vi "CRYPlot XY Graph.vi"(6 "sOption":string, 7 "pGraph VI In":refnum<vi>, 8 "sType":string, 9 "Flattened Property":string, 10 "Flattened Scale Property":string, 11 "Selected Rows In":i32[](array[numeric])) -> (0 "Color Info":u32[](array[numeric]), 1 "Curve Name":string[](array[string]), 2 "All Rows Out":i32[](array[numeric]), 3 "ItemSyms":i32[](array[numeric]))   [LabVIEW 2013]
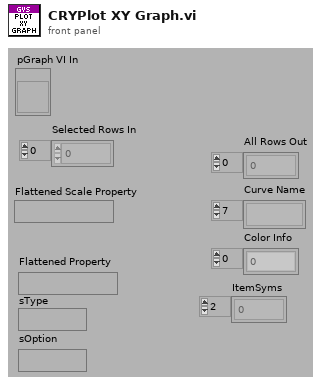
[diagram p1: front panel]
types:
  T1 = cluster{"Color":u32, "Interpolation":u8, "Point Style":u8, "Line Style":u8, "Point Color":u32, "Line Width":u8, "Bar Plot Style":u8, "Fill To":i16}[]
  T2 = typedef "CRYData Cluster.ctl" = cluster{"Name":string, "Curve":cluster{"x":dbl, "y":dbl, "z":dbl}[], "X data":u16, "Y data":u16, "Z data":u16, "X axis":u16, "Y axis":u16, "Z axis":u16, "X unit":string, "Y unit":string, "Z unit":string, "X dB ref":dbl, "Y dB ref":dbl, "Z dB ref":dbl, "single val":bool, "protected":bool, "display X":bool, "display Y":bool, "display Z":bool, "Test Info":string, "Step No.":i32, "Plot Settings":cluster{"Color":u32, "Interpolation":u8, "Point Style":u8, "Line Style":u8, "Point Color":u32, "Line Width":u8, "Bar Plot Style":u8, "Fill To":i16}, "AutoProtect":bool}
  T3 = cluster{"Color":u32, "Interpolation":u8, "Point Style":u8, "Line Style":u8, "Point Color":u32, "Line Width":u8, "Bar Plot Style":u8, "Fill To":i16}
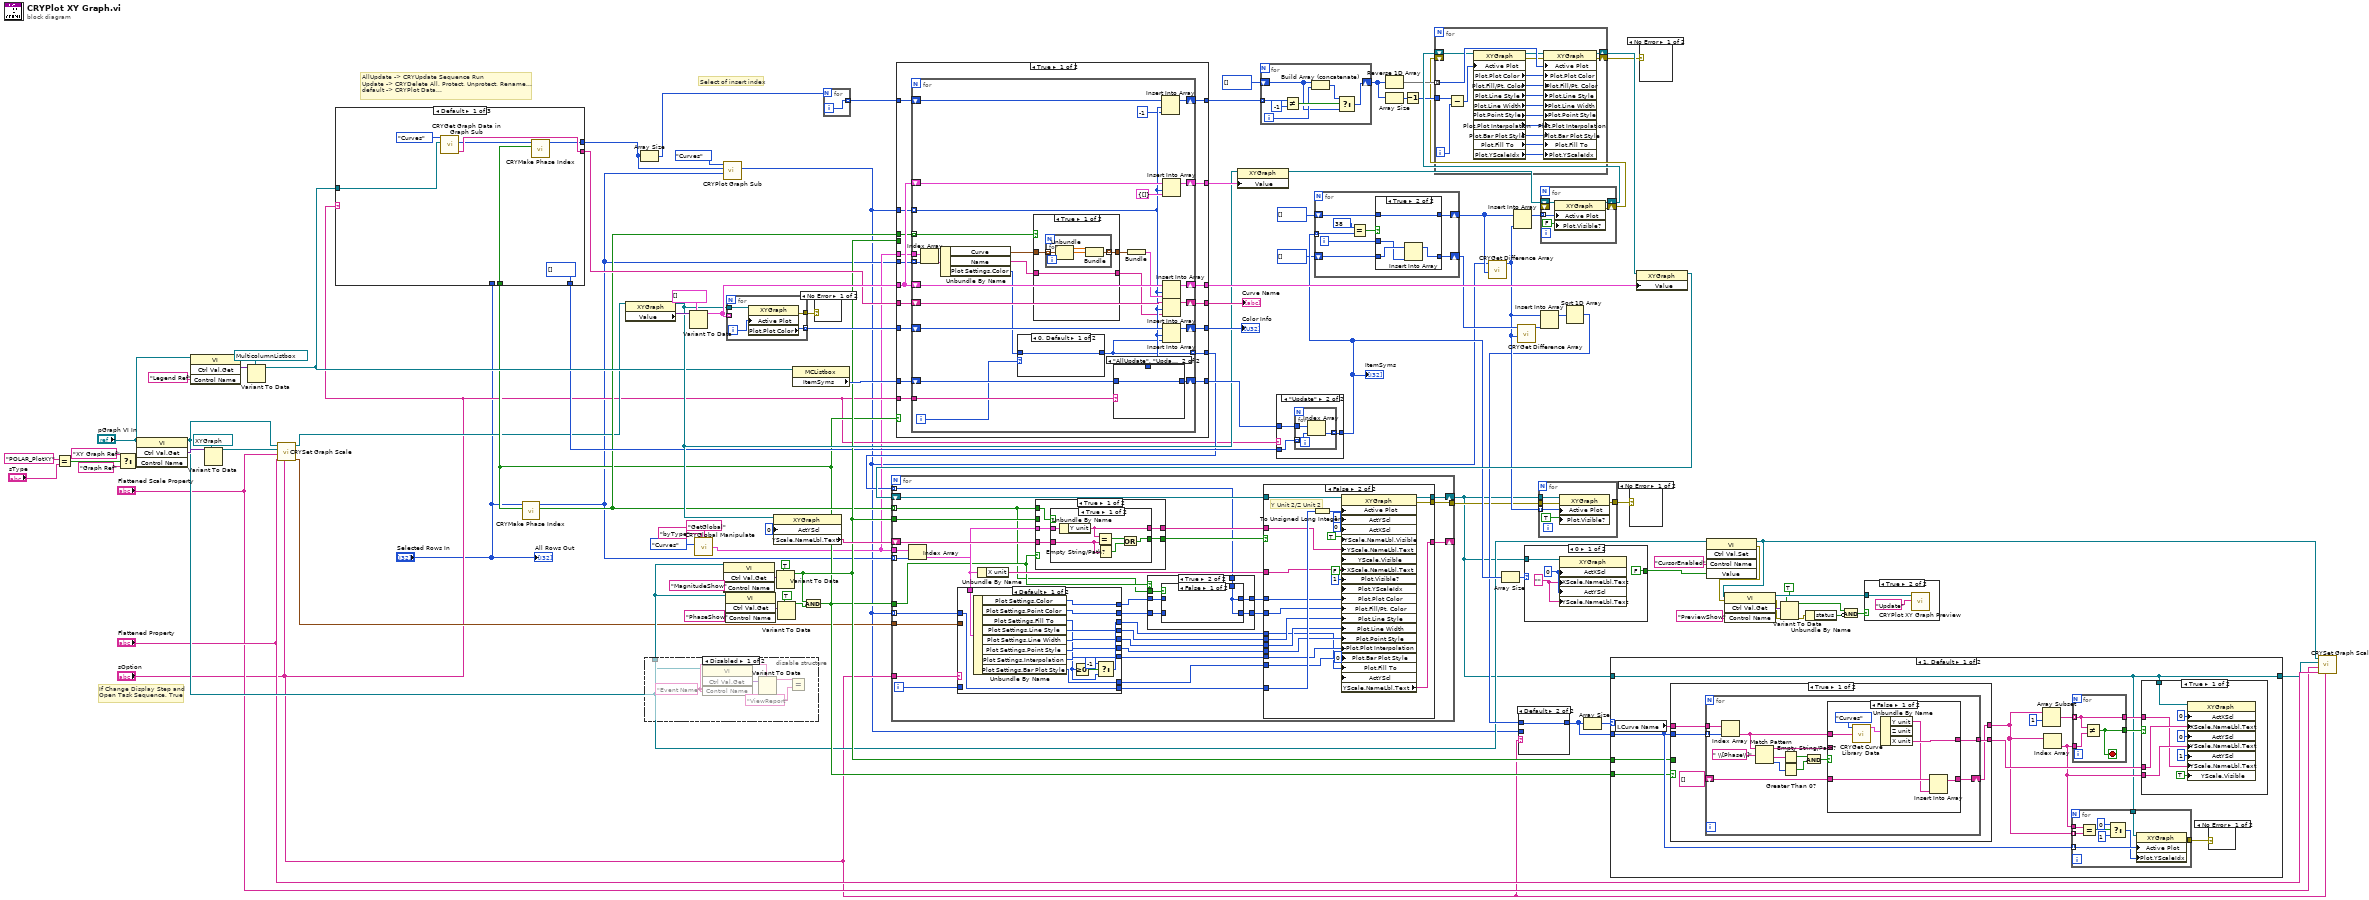
[diagram p0: block diagram]
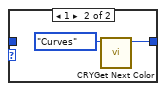
[diagram p5: hidden frame]
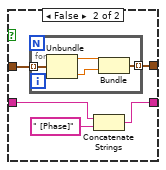
[diagram p6: hidden frame]
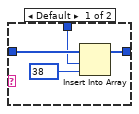
[diagram p7: hidden frame]
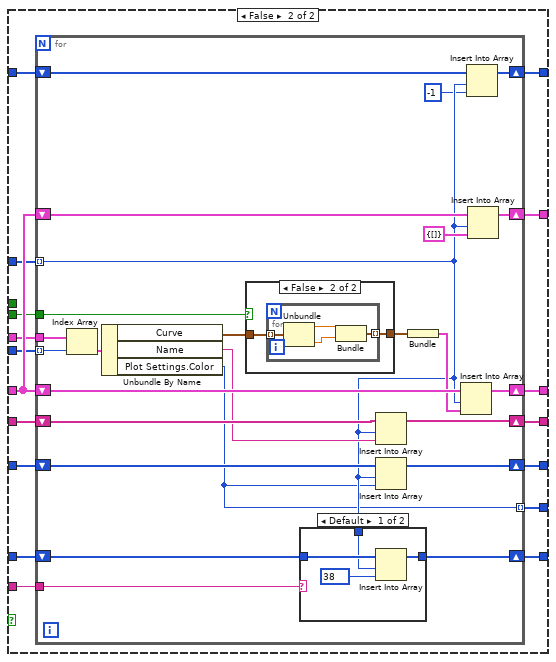
[diagram p8: hidden frame]
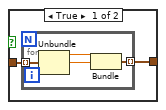
[diagram p9: hidden frame]
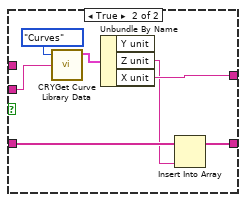
[diagram p14: hidden frame]
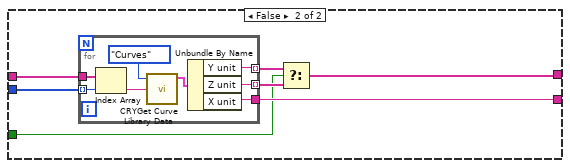
[diagram p15: hidden frame]
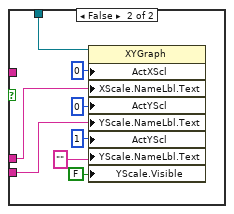
[diagram p16: hidden frame]
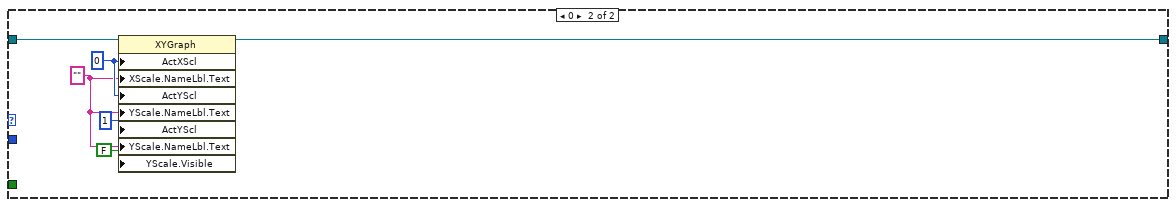
[diagram p17: hidden frame]
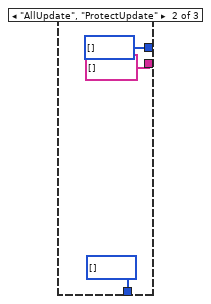
[diagram p19: hidden frame]
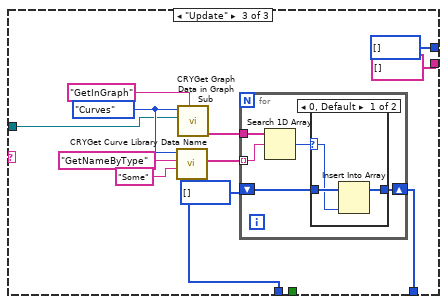
[diagram p20: hidden frame]
diagram:
  # "AllUpdate -> CRYUpdate Sequence Run\nUpdate -> CRYDelete All, Protect, Unprotect, Rename...\ndefault -> CRYPlot Data..."
  # "Select of insert index"
  # "If Change Display Step and \nOpen Task Sequence, True"
  n1 = Equal?(x="POLAR_PlotXY" ("Control Name"), y="sType") -> (x = y?=w33:bool)
  n2 = Select(t="XY Graph Ref", s=w33, f="Graph Ref" ("Control Name")) -> (s? t:f=w30:string)
  n3 = invoke class="VI" method="Ctrl Val.Get"(reference="pGraph VI In", "Control Name"=w30) -> (reference out=w19:refnum<vi>, "Get Control Value Variant"=w40:variant)  [unwired: 2 in, 2 out]
  n4 = invoke class="VI" method="Ctrl Val.Get"(reference="pGraph VI In", "Control Name"="Legend Ref") -> ("Get Control Value Variant"=w38:variant)  [unwired: 2 in, 3 out]
  n5 = Variant To Data(type=refnum<vi> refnum ("XY Graph"), Variant=w40) -> (data=w18:refnum<vi>)  [unwired: 1 in, 1 out]
  n6 = Variant To Data(type=refnum<vi> refnum ("GMListbox"), Variant=w38) -> (data=w35:refnum<vi>)  [unwired: 1 in, 1 out]
  n7 = call "CRYSet Graph Scale.vi"("sOption"="sOption", "Flattened Property"="Flattened Property", "Flattened Scale Property"="Flattened Scale Property", "pGraph In"=w18, "pGraph VI In"=w19) -> ("Plot Settings"=w16:T1, "pGraph Out"=w17:refnum<vi>)  [unwired: 5 in]
  n8 = property class="XYGraph"(reference=w17) -> (reference out=w59:refnum<vi>, "Value"=w97:variant)  [unwired: 1 in, 1 out]
  n9 = disable-structure shown="Disabled" {
    disable-tunnel: w19 -> [w101 _]
    frame Disabled {
      w102 = "Event Name" ("Control Name")
      n10 = invoke class="VI" method="Ctrl Val.Get"(reference=w101, "Control Name"=w102) -> ("Get Control Value Variant"=w105:variant)  [unwired: 2 in, 3 out]
      n11 = Variant To Data(type=w102, Variant=w105) -> (data=w104:string)  [unwired: 1 in, 1 out]
      n12 = Equal?(x=w104, y="ViewReport" ("regular expression")) -> ()  [unwired: 1 out]
    }
    frame Enabled {
    }
  }
  n13 = Variant To Data(type=cluster{cluster{"x":dbl, "z":dbl}[]}[] [], Variant=w97) -> (data=w96:cluster{cluster{"x":dbl, "z":dbl}[]}[])  [unwired: 1 in, 1 out]
  n14 = call "CRYGlobal Manipulate.vi"("Type"=enum16{"Curves", "Values", "Results", "WFM"}."Curves", "sOption"="byType", "sAction"="GetGlobal") -> ("Curves Out"=w6:T2[])  [unwired: 6 in, 6 out]
  n15 = invoke class="VI" method="Ctrl Val.Get"(reference=w19, "Control Name"="MagnitudeShow") -> ("Get Control Value Variant"=w69:variant)  [unwired: 2 in, 3 out]
  n16 = invoke class="VI" method="Ctrl Val.Get"(reference=w19, "Control Name"="PhaseShow") -> ("Get Control Value Variant"=w27:variant)  [unwired: 2 in, 3 out]
  n17 = for {
    tunnel: w96 -> [_] mode=indexing
    tunnel: w59 -> [w109]
    tunnel: [w108] -> w95 mode=indexing
    tunnel: [w106] -> w42
    i -> [w107]
    n18 = property class="XYGraph"(reference=w109, "Active Plot"=w107) -> (error out=w106:errorcluster, "Plot.Plot Color"=w108:u32)  [unwired: 1 in, 1 out]
  }
  n19 = property class="XYGraph"(reference=w59, "ActYScl"=0 ("Active Y Scale")) -> ("YScale.NameLbl.Text"=w58:string)  [unwired: 1 in, 2 out]
  n20 = Variant To Data(type=TRUE, Variant=w69) -> (data=w25:bool)  [unwired: 1 in, 1 out]
  n21 = Variant To Data(type=TRUE, Variant=w27) -> (data=w24:bool)  [unwired: 1 in, 1 out]
  n22 = property class="MCListbox"(reference=w35) -> ("ItemSyms"=w87:i32[])  [unwired: 1 in, 2 out]
  n23 = And(x=w25, y=w24) -> (x .and. y?=w20:bool)
  n24 = case shown="Default" "sOption" {
    tunnel: [w116 string[] [] ("Names Out") string[] [] ("Names Out")] -> w92
    tunnel: [w112 i32[] [] ("Rows") i32[] [] ("Rows")] -> w3
    tunnel: "Selected Rows In" -> [_ _ w125]
    tunnel: [i32[] [] i32[] [] w121] -> w23
    tunnel: w35 -> [w113 _ w120]
    tunnel: w20 -> [w111 _ _]
    frame Default {
      n25 = call "CRYGet Graph Data in Graph Sub.vi"("Legend Refnum"=w113, "Type In"=enum16{"Curves", "Values", "Results", "WFM"}."Curves" ("Type")) -> ("Names Out"=w116:string[], "Rows"=w110:i32[])  [unwired: 5 in, 3 out]
      n26 = call "CRYMake Phase Index.vi"("Mag_Phase Flag"=w111, "Selected Rows In"=w110) -> ("Selected Rows Out"=w112:i32[])  [unwired: 8 in, 1 out]
    }
    frame "AllUpdate", "ProtectUpdate" {
    }
    frame "Update" {
      w128 = enum16{"Curves", "Values", "Results", "WFM"}."Curves" ("Type")
      n27 = call "CRYGet Curve Library Data Name.vi"("nData"=w125, "sOption"="Some", "sAction"="GetNameByType", "Type"=w128) -> ("sNames"=w123:string[])  [unwired: 4 in, 3 out]
      n28 = call "CRYGet Graph Data in Graph Sub.vi"("sOption"="GetInGraph", "Legend Refnum"=w120, "Type In"=w128) -> ("Names Out"=w124:string[])  [unwired: 4 in, 4 out]
      n29 = for {
        tunnel: w124 -> [w133]
        tunnel: w123 -> [w132] mode=indexing
        shift-right: [w134] -> w121
        shift-left: i32[] [] -> [w135]
        n30 = Search 1D Array(1D array=w133, element=w132) -> (index of element=w136:i32)  [unwired: 1 in]
        n31 = case shown="0, Default" w136 {
          selector: w136 -> [w137 _]
          tunnel: w135 -> [w139 w140]
          tunnel: [w138 w140] -> w134
          frame 0, Default {
            n32 = Insert Into Array(array=w139, new element=w137) -> (w138:i32[])  [unwired: 1 in]
          }
          frame -1 {
          }
        }
      }
    }
  }
  n33 = call "CRYMake Phase Index.vi"("Mag_Phase Flag"=w20, "Selected Rows In"="Selected Rows In") -> ("Mag_Phase"=w22:bool[], "Selected Rows Out"=w2:i32[])  [unwired: 8 in]
  n34 = Array Size(array=w3) -> (size(s)=w65:i32)
  n35 = call "CRYPlot Graph Sub.vi"("nData2 In"=w2, "nData1 In"=w3, "Type"=enum16{"Curves", "Values", "Results", "WFM"}."Curves") -> ("nData Out"=w1:i32[])  [unwired: 8 in]
  n36 = case shown="No Error" w42 {
    frame No Error {
    }
    frame Error {
    }
  }
  n37 = for {
    N: w65 -> [_]
    tunnel: [w141] -> w85 mode=indexing
    i -> [w141]
  }
  n38 = case shown="True" w20 {
    tunnel: w96 -> [w158 w227]
    tunnel: w95 -> [w157 w226]
    tunnel: [w156 w225] -> w94
    tunnel: w92 -> [w155 w224]
    tunnel: [w154 w223] -> w89
    tunnel: [w153 w222] -> w88
    tunnel: w87 -> [w152 w221]
    tunnel: w85 -> [w151 w220]
    tunnel: [w150 w219] -> w84
    tunnel: [w149 w218] -> w75
    tunnel: [w148 w217] -> w62
    tunnel: w6 -> [w147 w216]
    tunnel: w2 -> [w146 w215]
    tunnel: w1 -> [w145 w214]
    tunnel: "sOption" -> [w144 w213]
    tunnel: w25 -> [_ w212]
    tunnel: w22 -> [w143 _]
    tunnel: [w142 w211] -> w21
    frame True {
      n39 = for {
        tunnel: w147 -> [w186]
        tunnel: w146 -> [w183] mode=indexing
        shift-right: [w184] -> w154
        shift-left: w158 -> [w185]
        tunnel: w145 -> [w167] mode=indexing
        shift-right: [w175] -> w156
        shift-left: w155 -> [w178]
        shift-right: [w176] -> w149
        shift-left: w157 -> [w177]
        shift-right: [w173] -> w153
        shift-left: w158 -> [w172]
        shift-right: [w170] -> w148
        shift-left: w152 -> [w171]
        shift-right: [w168] -> w150
        shift-left: w151 -> [w169]
        tunnel: w144 -> [w165]
        tunnel: w143 -> [w164] mode=indexing
        tunnel: [w159] -> w142 mode=indexing
        i -> [w161]
        n40 = Index Array(array=w186, index=w183) -> (element=w180:T2)
        n41 = Unbundle By Name(w180) -> ("Curve"=w181:cluster{"x":dbl, "y":dbl, "z":dbl}[], "Name"=w163:string, "Plot Settings.Color"=w160:u32)
        n42 = case shown="0, Default" w161 {
          tunnel: w160 -> [w187 _]
          tunnel: [w187 w188] -> w159
          frame 0, Default {
          }
          frame 1 {
            n43 = call "CRYGet Next Color.vi"("Type"=enum16{"Curves", "Values", "Results", "WFM"}."Curves") -> ("Color"=w188:u32)  [unwired: 10 out]
          }
        }
        n44 = case shown="True" w164 {
          tunnel: [w192 w201] -> w182
          tunnel: w181 -> [w191 w200]
          tunnel: w163 -> [w190 w199]
          tunnel: [w190 w197] -> w162
          frame True {
            n45 = for {
              tunnel: w191 -> [w196] mode=indexing
              tunnel: [w195] -> w192 mode=indexing
              n46 = Unbundle(w196) -> ("x"=w194:dbl, "y"=w193:dbl)  [unwired: 1 out]
              n47 = Bundle("x"=w194, "y"=w193) -> (w195:cluster{"x":dbl, "y":dbl})  [unwired: 1 out]
            }
          }
          frame False {
            n48 = for {
              tunnel: w200 -> [w205] mode=indexing
              tunnel: [w204] -> w201 mode=indexing
              n49 = Unbundle(w205) -> ("x"=w203:dbl, "z"=w202:dbl)  [unwired: 1 out]
              n50 = Bundle("x"=w203, "z"=w202) -> (w204:cluster{"x":dbl, "z":dbl})  [unwired: 1 out]
            }
            n51 = Concatenate Strings(w199, " [Phase]" ("regular expression")) -> (w197:string)
          }
        }
        n52 = case shown="\"AllUpdate\", \"Update\"" w165 {
          tunnel: w171 -> [w209 w210]
          tunnel: [w208 w210] -> w170
          tunnel: w167 -> [w206 _]
          frame Default {
            n53 = Insert Into Array(array=w209, index=w206, new element=38) -> (w208:i32[])
          }
          frame "AllUpdate", "Update" {
          }
        }
        n54 = Bundle(w182) -> (w179:cluster{cluster{"x":dbl, "z":dbl}[]})  [unwired: 1 in]
        n55 = Insert Into Array(array=w169, index=w167, new element=-1 ("new element/subarray")) -> (w168:i32[])
        n56 = Insert Into Array(array=w172, index=w167, new element=cluster{cluster{"x":dbl, "y":dbl}[]} {[]} ("output cluster")) -> (w173:cluster{cluster{"x":dbl, "z":dbl}[]}[])
        n57 = Insert Into Array(array=w185, index=w167, new element=w179) -> (w184:cluster{cluster{"x":dbl, "z":dbl}[]}[])
        n58 = Insert Into Array(array=w178, index=w167, new element=w162) -> (w175:string[])
        n59 = Insert Into Array(array=w177, index=w167, new element=w159) -> (w176:u32[])
      }
    }
    frame False {
      n60 = for {
        tunnel: w216 -> [w252]
        tunnel: w215 -> [w249] mode=indexing
        shift-right: [w250] -> w223
        shift-left: w227 -> [w251]
        tunnel: w214 -> [w232] mode=indexing
        shift-right: [w240] -> w225
        shift-left: w224 -> [w244]
        shift-right: [w241] -> w218
        shift-left: w226 -> [w242]
        shift-right: [w238] -> w222
        shift-left: w227 -> [w237]
        shift-right: [w235] -> w217
        shift-left: w221 -> [w236]
        shift-right: [w233] -> w219
        shift-left: w220 -> [w234]
        tunnel: w213 -> [w230]
        tunnel: w212 -> [w229]
        tunnel: [w228] -> w211 mode=indexing
        n61 = Index Array(array=w252, index=w249) -> (element=w246:T2)
        n62 = Unbundle By Name(w246) -> ("Curve"=w247:cluster{"x":dbl, "y":dbl, "z":dbl}[], "Name"=w243:string, "Plot Settings.Color"=w228:u32)
        n63 = case shown="False" w229 {
          tunnel: [w254 w260] -> w248
          tunnel: w247 -> [w253 w259]
          frame True {
            n64 = for {
              tunnel: w253 -> [w258] mode=indexing
              tunnel: [w257] -> w254 mode=indexing
              n65 = Unbundle(w258) -> ("x"=w256:dbl, "y"=w255:dbl)  [unwired: 1 out]
              n66 = Bundle("x"=w256, "y"=w255) -> (w257:cluster{"x":dbl, "y":dbl})  [unwired: 1 out]
            }
          }
          frame False {
            n67 = for {
              tunnel: w259 -> [w264] mode=indexing
              tunnel: [w263] -> w260 mode=indexing
              n68 = Unbundle(w264) -> ("x"=w262:dbl, "z"=w261:dbl)  [unwired: 1 out]
              n69 = Bundle("x"=w262, "z"=w261) -> (w263:cluster{"x":dbl, "z":dbl})  [unwired: 1 out]
            }
          }
        }
        n70 = case shown="Default" w230 {
          tunnel: w236 -> [w268 w269]
          tunnel: [w267 w269] -> w235
          tunnel: w232 -> [w265 _]
          frame Default {
            n71 = Insert Into Array(array=w268, index=w265, new element=38) -> (w267:i32[])
          }
          frame "AllUpdate", "Update" {
          }
        }
        n72 = Insert Into Array(array=w244, index=w232, new element=w243) -> (w240:string[])
        n73 = Insert Into Array(array=w242, index=w232, new element=w228) -> (w241:u32[])
        n74 = Bundle(w248) -> (w245:cluster{cluster{"x":dbl, "z":dbl}[]})  [unwired: 1 in]
        n75 = Insert Into Array(array=w251, index=w232, new element=w245) -> (w250:cluster{cluster{"x":dbl, "z":dbl}[]}[])
        n76 = Insert Into Array(array=w234, index=w232, new element=-1 ("new element/subarray")) -> (w233:i32[])
        n77 = Insert Into Array(array=w237, index=w232, new element=cluster{cluster{"x":dbl, "y":dbl}[]} {[]} ("output cluster")) -> (w238:cluster{cluster{"x":dbl, "z":dbl}[]}[])
      }
    }
  }
  "Curve Name" <- w94
  "Color Info" <- w75
  n78 = property class="XYGraph"(reference=w59, "Value"=w88) -> (reference out=w90:refnum<vi>)  [unwired: 1 in, 1 out]
  n79 = for {
    tunnel: w84 -> [w276] mode=indexing
    shift-right: [w272] -> w79
    shift-left: i32[] [] ("Selected Rows In") -> [w270]
    i -> [w271]
    n80 = Not Equal?(x=w276, y=-1) -> (x != y?=w274:bool)
    n81 = Build Array (concatenate)(w270, w271) -> (w273:i32[])
    n82 = Select(t=w273, s=w274, f=w270) -> (s? t:f=w272:i32[])
  }
  n83 = case shown="\"Update\"" "sOption" {
    tunnel: w23 -> [_ w279]
    tunnel: w62 -> [w277 w280]
    tunnel: [w277 w278] -> w61
    frame Default {
    }
    frame "Update" {
      n84 = for {
        tunnel: w280 -> [w283]
        tunnel: w279 -> [w282] mode=indexing
        tunnel: [w281] -> w278 mode=indexing
        n85 = Index Array(array=w283, index=w282) -> (element=w281:i32)
      }
    }
  }
  "ItemSyms" <- w61
  n86 = for {
    tunnel: w61 -> [w290] mode=indexing
    shift-right: [w289] -> w63
    shift-left: i32[] [] ("Selected Rows In") -> [w288]
    shift-right: [w284] -> w55
    shift-left: i32[] [] ("Selected Rows In") -> [w285]
    i -> [w287]
    n87 = Equal?(x=38, y=w290) -> (x = y?=w286:bool)
    n88 = case shown="True" w286 {
      tunnel: [w293 w299] -> w289
      tunnel: w288 -> [w294 w299]
      tunnel: w287 -> [w295 w297]
      tunnel: w285 -> [w292 w298]
      tunnel: [w292 w296] -> w284
      frame False {
        n89 = Insert Into Array(array=w294, new element=w295) -> (w293:i32[])  [unwired: 1 in]
      }
      frame True {
        n90 = Insert Into Array(array=w298, new element=w297) -> (w296:i32[])  [unwired: 1 in]
      }
    }
  }
  n91 = Reverse 1D Array(array=w79) -> (reversed array=w80:i32[])
  n92 = Array Size(array=w79) -> (size(s)=w78:i32)
  n93 = Decrement(x=w78) -> (x-1=w77:i32)
  n94 = call "CRYGet Difference Array.vi"("Array 2"=w63, "Array 1"=w1) -> ("Diff Out"=w54:i32[])  [unwired: 8 in, 1 out]
  n95 = Array Size(array=w61) -> (size(s)=w100:i32)
  n96 = Insert Into Array(array=w63, new element=w54) -> (w64:i32[])  [unwired: 1 in]
  n97 = call "CRYGet Difference Array.vi"("Array 2"=w54, "Array 1"=w55) -> ("Diff Out"=w53:i32[])  [unwired: 8 in, 1 out]
  n98 = for {
    shift-right: [w302] -> w82
    shift-left: w90 -> [w304]
    tunnel: w64 -> [w301] mode=indexing
    shift-right: [w300] -> w66
    shift-left: _ -> [_]
    n99 = property class="XYGraph"(reference=w304, "Active Plot"=w301, "Plot.Visible?"=FALSE ("Plot.Visible")) -> (reference out=w302:refnum<vi>, error out=w300:errorcluster)  [unwired: 1 in]
  }
  n100 = for {
    tunnel: w80 -> [w317] mode=indexing
    shift-right: [w315] -> w81
    shift-left: w82 -> [w316]
    tunnel: w77 -> [w312]
    shift-right: [w308] -> w76
    shift-left: w66 -> [_]
    i -> [w311]
    n101 = Subtract(x=w312, y=w311) -> (x-y=w310:i32)
    n102 = property class="XYGraph"(reference=w316, "Active Plot"=w310) -> (reference out=w314:refnum<vi>, error out=w309:errorcluster, "Plot.Plot Color"=w322:u32, "Plot.Fill/Pt. Color"=w321:u32, "Plot.Line Style"=w320:u8, "Plot.Line Width"=w319:u8, "Plot.Point Style"=w318:u8, "Plot.Plot Interpolation"=w313:u8, "Plot.Bar Plot Style"=w307:u8, "Plot.Fill To"=w306:i16, "Plot.YScaleIdx"=w305:u32)  [unwired: 1 in]
    n103 = property class="XYGraph"(reference=w314, error in=w309, "Active Plot"=w317, "Plot.Plot Color"=w322, "Plot.Fill/Pt. Color"=w321, "Plot.Line Style"=w320, "Plot.Line Width"=w319, "Plot.Point Style"=w318, "Plot.Plot Interpolation"=w313, "Plot.Bar Plot Style"=w307, "Plot.Fill To"=w306, "Plot.YScaleIdx"=w305) -> (reference out=w315:refnum<vi>, error out=w308:errorcluster)
  }
  n104 = Insert Into Array(array=w54, new element=w53) -> (w52:i32[])  [unwired: 1 in]
  n105 = Sort 1D Array(array=w52) -> (sorted array=w51:i32[])
  n106 = case shown="Default" "sOption" {
    tunnel: w51 -> [_ w324]
    tunnel: [w323 w324] -> w50
    tunnel: w1 -> [w323 _]
    frame "AllUpdate", "ProtectUpdate", "SepuenceOpen" {
    }
    frame Default {
    }
  }
  n107 = Array Size(array=w50) -> (size(s)=w57:i32)
  n108 = property class="XYGraph"(reference=w81, "Value"=w89) -> (reference out=w93:refnum<vi>)  [unwired: 1 in, 1 out]
  n109 = for {
    tunnel: w2 -> [w354] mode=indexing
    tunnel: w6 -> [w353]
    tunnel: w16 -> [w348]
    tunnel: "sOption" -> [w349]
    tunnel: w25 -> [w338]
    shift-right: [w350] -> w10
    shift-left: w93 -> [w337]
    tunnel: w1 -> [w336] mode=indexing
    shift-right: [w334] -> _
    shift-left: w58 -> [w341]
    tunnel: [w332] -> w43
    tunnel: w22 -> [w326] mode=indexing
    tunnel: w20 -> [w331]
    tunnel: w21 -> [w325] mode=indexing
    i -> [w342]
    n110 = Index Array(array=w353, index=w354) -> (element=w340:T2)
    n111 = case shown="Default" w349 {
      tunnel: w348 -> [_ w418]
      tunnel: [w408 w412] -> w330
      tunnel: [w407 w411] -> w328
      tunnel: [w406 w413] -> w347
      tunnel: [w405 w422] -> w346
      tunnel: [w404 w421] -> w345
      tunnel: [w403 w420] -> w344
      tunnel: [w402 w419] -> w343
      tunnel: w340 -> [w401 _]
      tunnel: w342 -> [_ w410]
      tunnel: [w397 w410] -> w335
      tunnel: w336 -> [w397 _]
      tunnel: [w396 w409] -> w333
      frame Default {
        n112 = Unbundle By Name(w401) -> ("Plot Settings.Color"=w408:u32, "Plot Settings.Point Color"=w407:u32, "Plot Settings.Fill To"=w398:i16, "Plot Settings.Line Style"=w405:u8, "Plot Settings.Line Width"=w404:u8, "Plot Settings.Point Style"=w403:u8, "Plot Settings.Interpolation"=w402:u8, "Plot Settings.Bar Plot Style"=w396:u8)
        n113 = Greater Or Equal To 0?(x=w398) -> (x >= 0?=w400:bool)
        n114 = Select(t=i16 -1 ("Fill To"), s=w400, f=w398) -> (s? t:f=w406:i16)
      }
      frame "SepuenceOpen" {
        n115 = Index Array(array=w418, index=w410) -> (element=w417:T3)
        n116 = Unbundle By Name(w417) -> ("Color"=w412:u32, "Point Color"=w411:u32, "Fill To"=w414:i16, "Line Style"=w422:u8, "Line Width"=w421:u8, "Point Style"=w420:u8, "Interpolation"=w419:u8, "Bar Plot Style"=w409:u8)
        n117 = Greater Or Equal To 0?(x=w414) -> (x >= 0?=w416:bool)
        n118 = Select(t=i16 -1 ("Fill To"), s=w416, f=w414) -> (s? t:f=w413:i16)
      }
    }
    n119 = Unbundle By Name(w340) -> ("X unit"=w339:string)
    n120 = case shown="True" w331 {
      tunnel: [w370 w385] -> w352
      tunnel: [w369 w384] -> w351
      tunnel: w341 -> [w368 w383]
      tunnel: w340 -> [w367 w382]
      tunnel: w338 -> [_ w381]
      tunnel: w326 -> [w366 _]
      frame True {
        n121 = case shown="True" w366 {
          tunnel: [w371 w377] -> w370
          tunnel: [w375 w380] -> w369
          tunnel: w368 -> [w374 w378]
          tunnel: w367 -> [w376 w379]
          frame True {
            n122 = Unbundle By Name(w376) -> ("Y unit"=w375:string)
            n123 = Equal?(x=w375, y=w374) -> (x = y?=w372:bool)
            n124 = Empty String/Path?(string/path=w374) -> (empty?=w373:bool)
            n125 = Or(x=w372, y=w373) -> (x .or. y?=w371:bool)
          }
          frame False {
            n126 = Unbundle By Name(w379) -> ("Z unit"=w380:string)
            n127 = Equal?(x=w380, y=w378) -> (x = y?=w377:bool)
          }
        }
      }
      frame False {
        n128 = case shown="False" w381 {
          tunnel: [w386 w392] -> w385
          tunnel: [w390 w395] -> w384
          tunnel: w383 -> [w389 w393]
          tunnel: w382 -> [w391 w394]
          frame True {
            n129 = Unbundle By Name(w391) -> ("Y unit"=w390:string)
            n130 = Equal?(x=w390, y=w389) -> (x = y?=w387:bool)
            n131 = Empty String/Path?(string/path=w389) -> (empty?=w388:bool)
            n132 = Or(x=w387, y=w388) -> (x .or. y?=w386:bool)
          }
          frame False {
            n133 = Unbundle By Name(w394) -> ("Z unit"=w395:string)
            n134 = Equal?(x=w395, y=w393) -> (x = y?=w392:bool)
          }
        }
      }
    }
    n135 = case shown="True" w331 {
      tunnel: w330 -> [w356 w360]
      tunnel: [w356 w361] -> w329
      tunnel: w328 -> [w355 w358]
      tunnel: [w355 w359] -> w327
      tunnel: w326 -> [_ w362]
      tunnel: w325 -> [_ w357]
      frame False {
      }
      frame True {
        n136 = case shown="False" w362 {
          tunnel: [w363 w365] -> w361
          tunnel: w360 -> [_ w365]
          tunnel: [w363 w364] -> w359
          tunnel: w358 -> [_ w364]
          tunnel: w357 -> [w363 _]
          frame False {
          }
          frame True {
          }
        }
      }
    }
    n137 = case shown="False" w352 {
      tunnel: w339 -> [w432 w442]
      tunnel: w337 -> [w440 w461]
      tunnel: w335 -> [w439 w462]
      tunnel: w351 -> [w427 w447]
      tunnel: [w438 w460] -> w350
      tunnel: w329 -> [w437 w459]
      tunnel: w327 -> [w425 w458]
      tunnel: w347 -> [w424 w443]
      tunnel: w346 -> [w436 w457]
      tunnel: w345 -> [w435 w456]
      tunnel: w344 -> [w434 w455]
      tunnel: w343 -> [w433 w454]
      tunnel: [w427 w445] -> w334
      tunnel: w333 -> [w426 w444]
      tunnel: [w423 w441] -> w332
      frame True {
        w429 = 0 ("Active X Scale")
        # "Y Unit 1/Z Unit 1"
        n138 = To Unsigned Long Integer(number=w439) -> (unsigned 32bit integer=w428:u32)
        n139 = property class="XYGraph"(reference=w440, "Active Plot"=w428, "ActXScl"=w429, "XScale.NameLbl.Text"=w432, "ActYScl"=w429, "YScale.NameLbl.Text"=w427, "Plot.Visible?"=FALSE ("Plot.Visible"), "Plot.YScaleIdx"=u32 0 ("Plot.Y Scale Index"), "Plot.Plot Color"=w437, "Plot.Fill/Pt. Color"=w425, "Plot.Line Style"=w436, "Plot.Line Width"=w435, "Plot.Point Style"=w434, "Plot.Plot Interpolation"=w433, "Plot.Bar Plot Style"=w426, "Plot.Fill To"=w424) -> (reference out=w438:refnum<vi>, error out=w423:errorcluster)  [unwired: 1 in]
      }
      frame False {
        w450 = TRUE ("Y Scale.Name Label.Visible")
        # "Y Unit 2/Z Unit 2"
        n140 = To Unsigned Long Integer(number=w462) -> (unsigned 32bit integer=w449:u32)
        n141 = property class="XYGraph"(reference=w461, "Active Plot"=w449, "ActYScl"=1 ("Active Y Scale"), "ActXScl"=0 ("Active X Scale"), "YScale.NameLbl.Visible"=w450, "YScale.NameLbl.Text"=w447, "YScale.Visible"=w450, "XScale.NameLbl.Text"=w442, "Plot.Visible?"=FALSE ("Plot.Visible"), "Plot.YScaleIdx"=u32 1 ("Plot.Y Scale Index"), "Plot.Plot Color"=w459, "Plot.Fill/Pt. Color"=w458, "Plot.Line Style"=w457, "Plot.Line Width"=w456, "Plot.Point Style"=w455, "Plot.Plot Interpolation"=w454, "Plot.Bar Plot Style"=w444, "Plot.Fill To"=w443, "ActYScl"=0 ("Active Y Scale")) -> (reference out=w460:refnum<vi>, error out=w441:errorcluster, "YScale.NameLbl.Text"=w445:string)  [unwired: 1 in]
      }
    }
  }
  n142 = case shown="0" w100 {
    tunnel: w10 -> [w464 _]
    tunnel: [FALSE TRUE] -> w99
    frame 0 {
      w466 = 0 ("Active X Scale")
      w465 = "" ("X Scale.Name Label.Text")
      n143 = property class="XYGraph"(reference=w464, "ActXScl"=w466, "XScale.NameLbl.Text"=w465, "ActYScl"=w466, "YScale.NameLbl.Text"=w465) -> ()  [unwired: 1 in, 2 out]
    }
    frame 1, Default {
    }
  }
  n144 = for {
    tunnel: w10 -> [w472]
    tunnel: w54 -> [w470] mode=indexing
    tunnel: [w469] -> w67
    tunnel: w43 -> [w468]
    n145 = property class="XYGraph"(reference=w472, error in=w468, "Active Plot"=w470, "Plot.Visible?"=TRUE ("Plot.Visible")) -> (error out=w469:errorcluster)  [unwired: 1 out]
  }
  n146 = case shown="1, Default" w57 {
    tunnel: w50 -> [w477 _]
    tunnel: w10 -> [w473 w565]
    tunnel: w25 -> [w476 _]
    tunnel: w20 -> [w474 _]
    tunnel: [w473 w561] -> w11
    frame 1, Default {
      n147 = local read "Curve Name"() -> (w485:string[])
      n148 = case shown="True" w474 {
        tunnel: w485 -> [w490 w524]
        tunnel: [w489 w521] -> w481
        tunnel: [w486 w520] -> w479
        tunnel: w477 -> [w488 w519]
        tunnel: w476 -> [_ w518]
        frame True {
          n149 = for {
            tunnel: w490 -> [w502]
            tunnel: w488 -> [w503] mode=indexing
            tunnel: [w500] -> w489
            shift-right: [w501] -> w486
            shift-left: string[] [] -> [w491]
            n150 = Index Array(array=w502, index=w503) -> (element=w499:string)
            n151 = Match Pattern(string=w499, regular expression=" \\[Phase\\]") -> (before substring=w492:string, after substring=w497:string, offset past match=w496:i32)  [unwired: 1 in, 1 out]
            n152 = Empty String/Path?(string/path=w497) -> (empty?=w494:bool)
            n153 = Greater Than 0?(x=w496) -> (x > 0?=w493:bool)
            n154 = And(x=w494, y=w493) -> (x .and. y?=w495:bool)
            n155 = case shown="False" w495 {
              tunnel: [w505 w512] -> w501
              tunnel: [w508 w515] -> w500
              tunnel: w499 -> [w507 _]
              tunnel: w492 -> [_ w514]
              tunnel: w491 -> [w506 w513]
              frame False {
                n156 = call "CRYGet Curve Library Data.vi"("Type"=enum16{"Curves", "Values", "Results", "WFM"}."Curves", "Data Name"=w507) -> ("Curve"=w509:T2)  [unwired: 4 out]
                n157 = Unbundle By Name(w509) -> ("Y unit"=w504:string, "X unit"=w508:string)  [unwired: 1 out]
                n158 = Insert Into Array(array=w506, new element=w504) -> (w505:string[])  [unwired: 1 in]
              }
              frame True {
                n159 = call "CRYGet Curve Library Data.vi"("Type"=enum16{"Curves", "Values", "Results", "WFM"}."Curves", "Data Name"=w514) -> ("Curve"=w516:T2)  [unwired: 4 out]
                n160 = Unbundle By Name(w516) -> ("Z unit"=w511:string, "X unit"=w515:string)  [unwired: 1 out]
                n161 = Insert Into Array(array=w513, new element=w511) -> (w512:string[])  [unwired: 1 in]
              }
            }
          }
        }
        frame False {
          n162 = for {
            tunnel: w524 -> [w531]
            tunnel: w519 -> [w532] mode=indexing
            tunnel: [w527] -> w523 mode=indexing
            tunnel: [w526] -> w522 mode=indexing
            tunnel: [w525] -> w521
            n163 = Index Array(array=w531, index=w532) -> (element=w530:string)
            n164 = call "CRYGet Curve Library Data.vi"("Type"=enum16{"Curves", "Values", "Results", "WFM"}."Curves", "Data Name"=w530) -> ("Curve"=w528:T2)  [unwired: 4 out]
            n165 = Unbundle By Name(w528) -> ("Y unit"=w527:string, "Z unit"=w526:string, "X unit"=w525:string)
          }
          n166 = Select(t=w523, s=w518, f=w522) -> (s? t:f=w520:string[])
        }
      }
      n167 = Array Subset(array=w479, index=1) -> (w483:string[])  [unwired: 1 in]
      n168 = Index Array(array=w479) -> (element=w478:string)  [unwired: 1 in]
      n169 = for {
        tunnel: w477 -> [w541] mode=indexing
        tunnel: w479 -> [w539] mode=indexing
        tunnel: w478 -> [w540]
        tunnel: w473 -> [w534]
        tunnel: [w533] -> w475
        n170 = Equal?(x=w540, y=w539) -> (x = y?=w538:bool)
        n171 = Select(t=u32 0 ("Plot.Y Scale Index"), s=w538, f=u32 1 ("Plot.Y Scale Index")) -> (s? t:f=w535:u32)
        n172 = property class="XYGraph"(reference=w534, "Active Plot"=w541, "Plot.YScaleIdx"=w535) -> (error out=w533:errorcluster)  [unwired: 1 in, 1 out]
      }
      n173 = for {
        tunnel: w483 -> [w558] mode=indexing
        tunnel: w478 -> [w560]
        tunnel: [w559] -> w482
        tunnel: [w558] -> w480
        stop <- w559 stop-if-true
        n174 = Not Equal?(x=w558, y=w560) -> (x != y?=w559:bool)
      }
      n175 = case shown="True" w482 {
        tunnel: w473 -> [w547 w555]
        tunnel: w478 -> [w545 w553]
        tunnel: w481 -> [w544 w551]
        tunnel: w480 -> [w542 _]
        frame True {
          n176 = property class="XYGraph"(reference=w547, "ActXScl"=0 ("Active X Scale"), "XScale.NameLbl.Text"=w544, "ActYScl"=0 ("Active X Scale"), "YScale.NameLbl.Text"=w545, "ActYScl"=1 ("Active Y Scale"), "YScale.NameLbl.Text"=w542, "YScale.Visible"=TRUE ("Y Scale.Visible")) -> ()  [unwired: 1 in, 2 out]
        }
        frame False {
          n177 = property class="XYGraph"(reference=w555, "ActXScl"=0 ("Active X Scale"), "XScale.NameLbl.Text"=w551, "ActYScl"=0 ("Active X Scale"), "YScale.NameLbl.Text"=w553, "ActYScl"=1 ("Active Y Scale"), "YScale.NameLbl.Text"="" ("Y Scale.Name Label.Text"), "YScale.Visible"=FALSE ("Y Scale.Visible")) -> ()  [unwired: 1 in, 2 out]
        }
      }
      n178 = case shown="No Error" w475 {
        frame No Error {
        }
        frame Error {
        }
      }
    }
    frame 0 {
      w566 = 0 ("Active X Scale")
      w563 = "" ("X Scale.Name Label.Text")
      n179 = property class="XYGraph"(reference=w565, "ActXScl"=w566, "XScale.NameLbl.Text"=w563, "ActYScl"=w566, "YScale.NameLbl.Text"=w563, "ActYScl"=1 ("Active Y Scale"), "YScale.NameLbl.Text"=w563, "YScale.Visible"=FALSE ("Y Scale.Visible")) -> (reference out=w561:refnum<vi>)  [unwired: 1 in, 1 out]
    }
  }
  n180 = case shown="No Error" w67 {
    frame No Error {
    }
    frame Error {
    }
  }
  n181 = case shown="No Error" w76 {
    frame No Error {
    }
    frame Error {
    }
  }
  n182 = invoke class="VI" method="Ctrl Val.Set"(reference=w19, "Control Name"="CursorEnabled", "Value"=w99) -> (reference out=w15:refnum<vi>, error out=w49:errorcluster)  [unwired: 2 in, 3 out]
  n183 = invoke class="VI" method="Ctrl Val.Get"(reference=w15, error in=w49, "Control Name"="PreviewShow") -> (reference out=w73:refnum<vi>, error out=w48:errorcluster, "Get Control Value Variant"=w72:variant)  [unwired: 1 in, 1 out]
  n184 = Variant To Data(error in=w48, type=TRUE, Variant=w72) -> (data=w46:bool, error out=w47:errorcluster)
  n185 = Unbundle By Name(w47) -> ("status"=w45:bool)
  n186 = Compound Arithmetic op=AND(w46, invert w45) -> (w44:bool)
  n187 = case shown="True" w44 {
    tunnel: w73 -> [_ w568]
    frame False {
    }
    frame True {
      n188 = call "CRYPlot XY Graph Preview.vi"("sOption"="Update", "Graph VI Ref"=w568) -> ()  [unwired: 10 in]
    }
  }
  n189 = call "CRYSet Graph Scale.vi"("sOption"="sOption", "Flattened Property"="Flattened Property", "Flattened Scale Property"="Flattened Scale Property", "pGraph In"=w11, "pGraph VI In"=w15) -> ()  [unwired: 5 in, 2 out]
  "All Rows Out" <- "Selected Rows In"
